vi "CameraAcq.vi"() -> ()   [LabVIEW 2023]
uses:
  <vilib>/vision/driver/NI_Vision_Acquisition_Software.lvlib
  <vilib>/userDefined/High Color/IMAQdx.ctl
panel:
  in  "Boolean":bool
  out "Image2":T1(plugin-control)
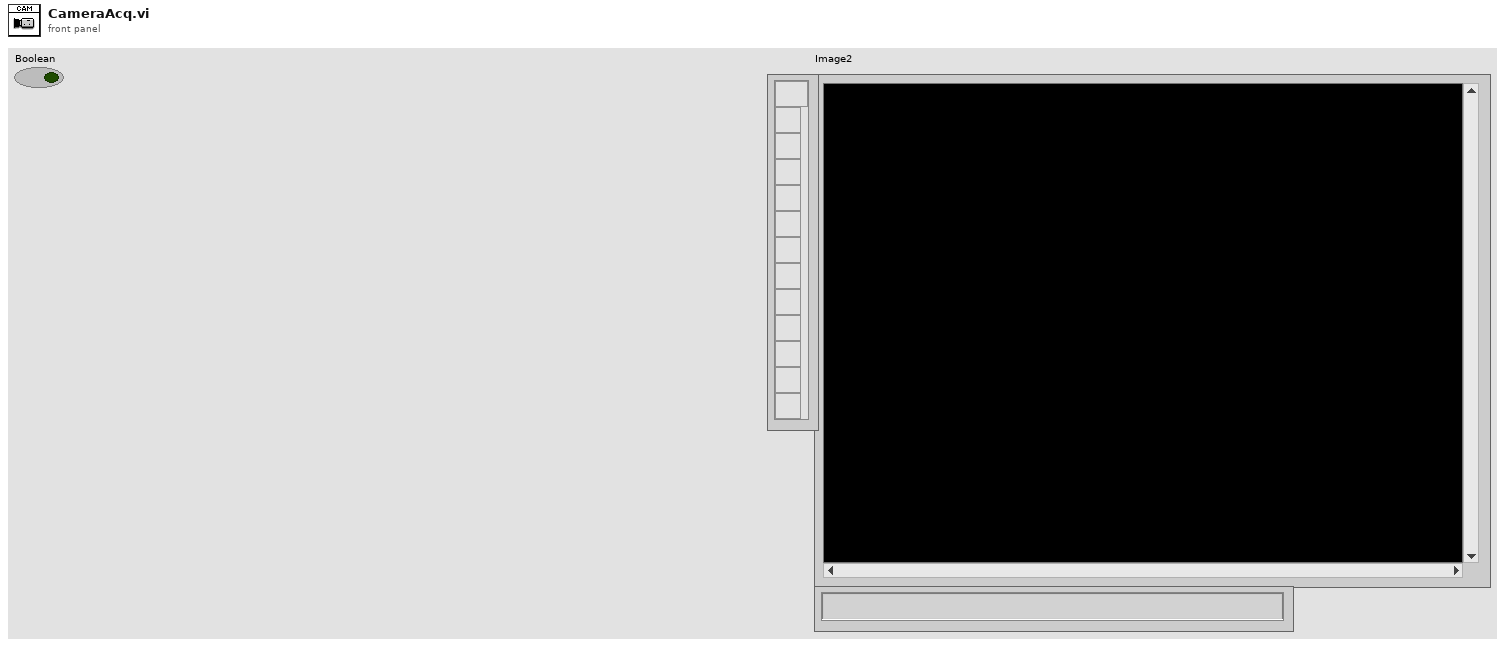
[diagram p1: front panel]
types:
  T1 = typedef "IMAQ Image.ctl" = refnum<image>
  T2 = typedef "IMAQdx.ctl" = refnum<k21>
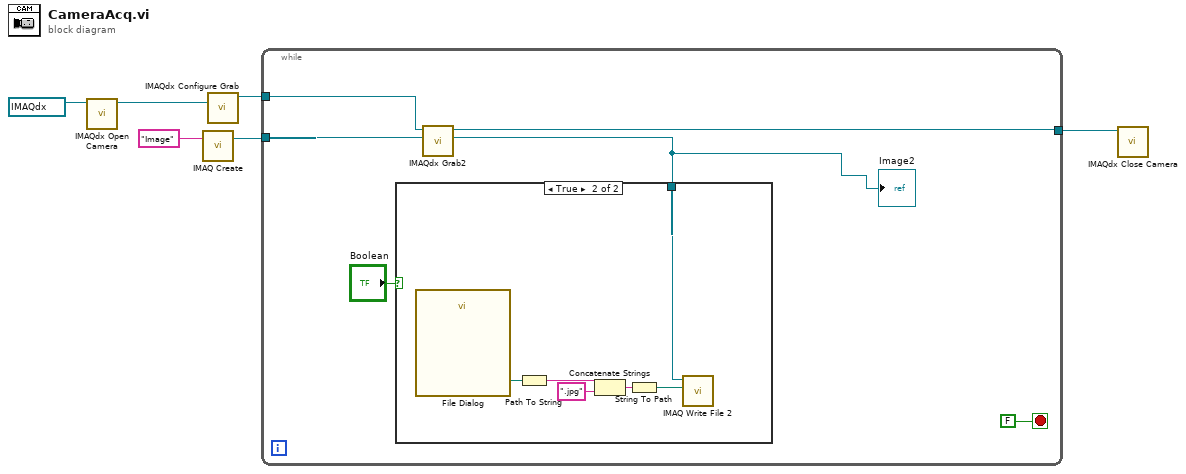
[diagram p0: block diagram]
diagram:
  n1 = call <vilib>:"IMAQdx Open Camera.vi"("Session In"=T2 "cam0") -> ("Session Out"=w3:T2)  [unwired: 9 in, 1 out]
  n2 = call "IMAQ Create"("Image Name"="Image") -> ("New Image"=w6:T1)  [unwired: 4 in, 1 out]
  n3 = call <vilib>:"IMAQdx Configure Grab.vi"("Session In"=w3) -> ("Session Out"=w2:T2)  [unwired: 9 in, 1 out]
  n4 = while {
    tunnel: w2 -> [w12]
    tunnel: w6 -> [w11]
    tunnel: [w10] -> w4
    stop <- FALSE stop-if-true
    n5 = call <vilib>:"IMAQdx Grab2.vi"("Image In"=w11, "Session In"=w12) -> ("Image Out"=w9:T1, "Session Out"=w10:T2)  [unwired: 6 in, 2 out]
    "Image2" <- w9
    n6 = case shown="True" "Boolean" {
      tunnel: w9 -> [_ w18]
      frame False {
      }
      frame True {
        n7 = call "File Dialog"() -> ("selected path"=w17:path)  [unwired: 12 in, 3 out]
        n8 = Path To String(path=w17) -> (string=w16:string)
        n9 = Concatenate Strings(w16, ".jpg" ("string")) -> (w14:string)
        n10 = String To Path(string=w14) -> (path=w13:path)
        n11 = call-poly "IMAQ Write File 2"("File Path"=w13, "Image"=w18) -> ()  [unwired: 8 in, 2 out]
      }
    }
  }
  n12 = call <vilib>:"IMAQdx Close Camera.vi"("Session In"=w4) -> ()  [unwired: 10 in, 1 out]
